vi "Back EMF FPGA Voltage to Voltage.vi"(11 "Back EMF In":i16) -> (3 "Back EMF Out":dbl)   [LabVIEW 2018]
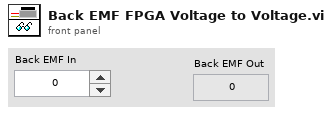
[diagram p1: front panel]
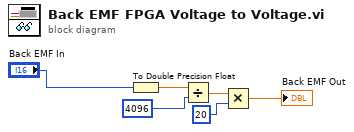
[diagram p0: block diagram]
diagram:
  n1 = To Double Precision Float(number="Back EMF In") -> (double precision float=w6:dbl)
  n2 = Divide(x=w6, y=4096) -> (x/y=w4:dbl)
  n3 = Multiply(x=w4, y=20) -> (x*y=→"Back EMF Out":dbl)
